vi "MVP Valve Read.vi"(0 "VISA resource name":refnum<visa-resource-name>="COM1", 11 "error in (no error)":errorcluster) -> (4 "VISA resource name out":refnum<visa-resource-name>, 8 "Output String":string, 15 "error out":errorcluster)   [LabVIEW 2015]
doc: "Reads a response from the pump affter a command is sent\n\nModified from original which is Copyright 2005, National Instruments Corporation"
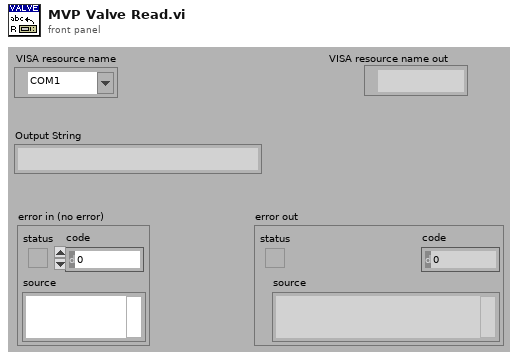
[diagram p1: front panel]
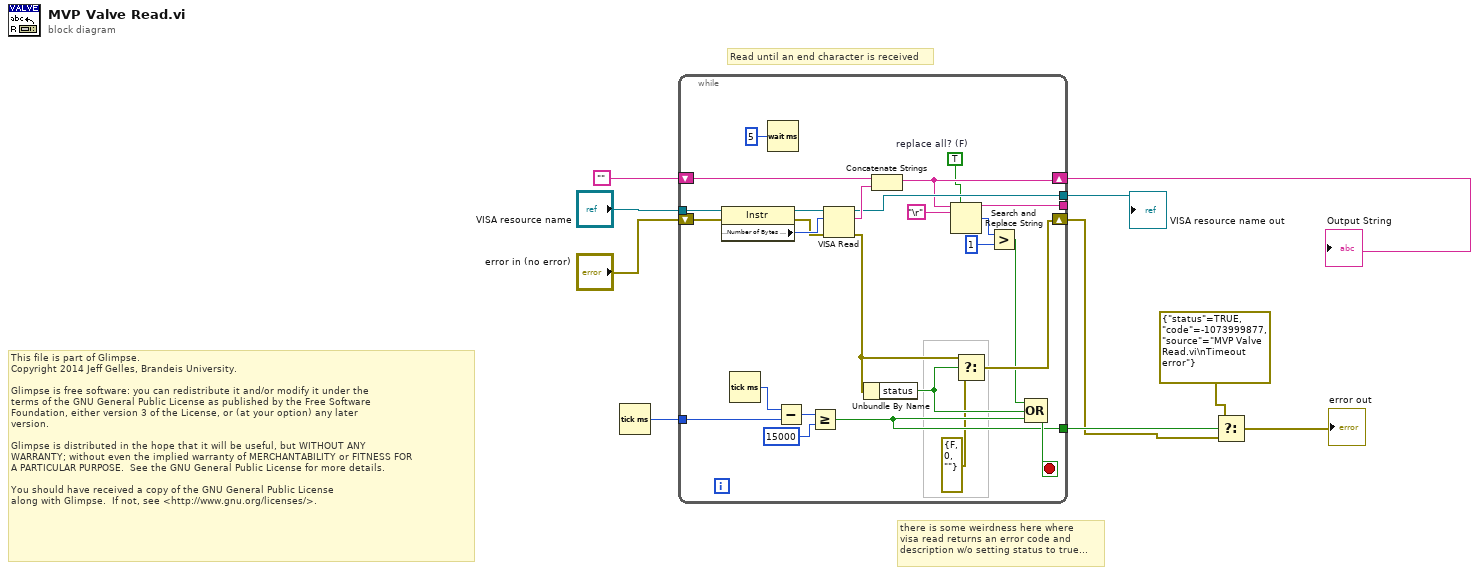
[diagram p0: block diagram]
diagram:
  # "This file is part of Glimpse. \nCopyright 2014 Jeff Gelles, Brandeis University.    \n\nGlimpse is free software: you can redistribute it and/or modify it under the \nterms of the GNU General Public License as published by the Free Software \nFoundation, either version 3 of the License, or (at your option) any later \nversion.\n\nGlimpse is distributed in the hope that it will be useful, but WITHOUT ANY \nWARRANTY; without even the implied warranty of MERCHANTABILITY or FITNESS FOR \nA PARTICULAR PURPOSE.  See the GNU General Public License for more details.\n\nYou should have received a copy of the GNU General Public License\nalong with Glimpse.  If not, see <http://www.gnu.org/licenses/>."
  # "there is some weirdness here where \nvisa read returns an error code and\ndescription w/o setting status to true..."
  # "Read until an end character is received"
  n1 = Tick Count (ms)() -> (millisecond timer value=w7:u32)
  n2 = while {
    tunnel: "VISA resource name" -> [w36]
    shift-right: [w17] -> w2
    shift-left: "" -> [w30]
    tunnel: [w29] -> w4
    tunnel: w7 -> [w26]
    tunnel: [w22] -> w6
    shift-right: [w18] -> w5
    shift-left: "error in (no error)" -> [w32]
    tunnel: [w14] -> _
    stop <- w23 stop-if-true
    w11 = TRUE  # replace all? (F)
    n3 = property class="Instr"(reference=w36, error in=w32) -> (reference out=w34:refnum<visa-resource-name>, error out=w33:errorcluster, "Serial Settings:Number of Bytes at Serial Port"=w35:u32)
    n4 = Tick Count (ms)() -> (millisecond timer value=w27:u32)
    n5 = Wait (ms)(milliseconds to wait=u32 5) -> ()  [unwired: 1 out]
    n6 = Subtract(x=w27, y=w26) -> (x-y=w25:u32)
    n7 = Greater Or Equal?(x=w25, y=u32 15000) -> (x >= y?=w22:bool)
    n8 = VISA Read(VISA resource name=w34, byte count=w35, error in (no error)=w33) -> (VISA resource name out=w29:refnum<visa-resource-name>, read buffer=w31:string, error out=w20:errorcluster)  [unwired: 1 out]
    n9 = Unbundle By Name(w20) -> ("status"=w21:bool)
    n10 = Concatenate Strings(w30, w31) -> (w17:string)
    n11 = Search and Replace String(replace all?=w11, input string=w17, search string="\r") -> (result string=w14:string, number of replacements=w13:i32)  [unwired: 1 in, 6 out]
    n12 = Select(t=w20, s=w21, f=errorcluster {"status"=FALSE, "code"=0, "source"=""}) -> (s? t:f=w18:errorcluster)
    n13 = Greater?(x=w13, y=1) -> (0:w15:bool)
    n14 = Compound Arithmetic op=OR(w15, w21, w22) -> (w23:bool)
  }
  "Output String" <- w2
  "VISA resource name out" <- w4
  n15 = Select(t=errorcluster {"status"=TRUE, "code"=-1073999877, "source"="MVP Valve Read.vi\nTimeout error"}, s=w6, f=w5) -> (s? t:f=→"error out":errorcluster)
